vi "Write Timeout Event.vi"(8 "error in (no error)":errorcluster, 10 "Timeout Event":bool, 11 "AnalogInput in":refnum<class "AnalogInput.lvclass">) -> (0 "error out":errorcluster, 3 "AnalogInput out":refnum<class "AnalogInput.lvclass">)   [LabVIEW 2019, in "AnalogInput.lvlib" / "AnalogInput.lvclass"]
uses:
  Library/AnalogInput.lvclass
  Library/AnalogInput.lvclass/AnalogInput.ctl
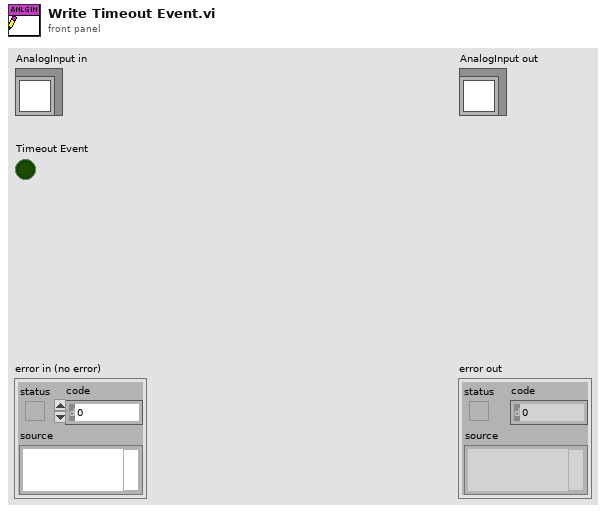
[diagram p1: front panel]
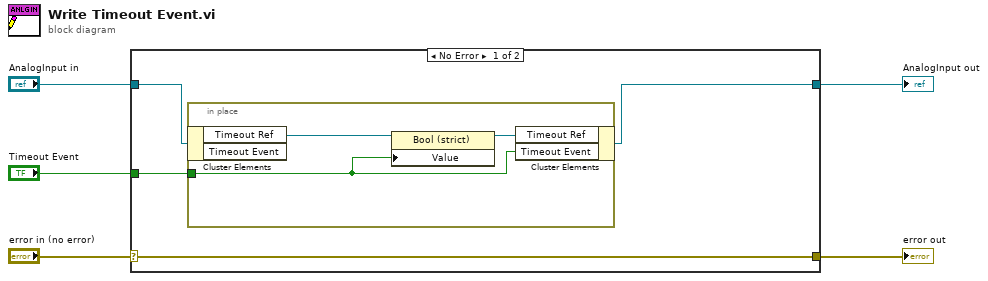
[diagram p0: block diagram]
diagram:
  n1 = case shown="No Error" "error in (no error)" {
    selector: "error in (no error)" -> [w9 w13]
    tunnel: [w9 w13] -> w4
    tunnel: [w6 w14] -> w2
    tunnel: "AnalogInput in" -> [w8 w14]
    tunnel: "Timeout Event" -> [w7 _]
    frame No Error {
      n2 = in-place {
        in-place-border: w7 -> [w10]
        n3 = in-place-cluster #1(w8) -> ("Timeout Ref"=w12:refnum<vi>)  [unwired: 1 out]
        n4 = property class="Bool (strict)"(reference=w12, "Value"=w10) -> (reference out=w11:refnum<vi>)  [unwired: 1 in, 1 out]
        n5 = in-place-cluster #1("Timeout Ref"=w11, "Timeout Event"=w10) -> (w6:refnum<class "AnalogInput.lvclass">)
      }
    }
    frame Error {
    }
  }
  "error out" <- w4
  "AnalogInput out" <- w2
